vi "Test Disk Space Monitor.vi"() -> ()   [LabVIEW 2020]
uses:
  DiskSpaceMonitor/DiskSpaceMonitor.xctl
panel:
  in  "DiskSpaceMonitor":dbl(xcontrol)
  in  "stop":bool
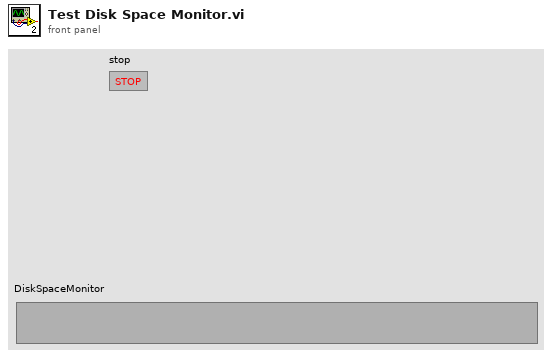
[diagram p1: front panel]
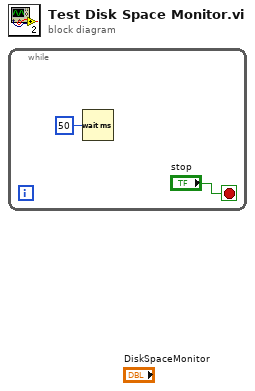
[diagram p0: block diagram]
diagram:
  n1 = while {
    stop <- "stop" stop-if-true
    n2 = Wait (ms)(milliseconds to wait=u32 50) -> ()  [unwired: 1 out]
  }
